vi "DCA Calibration Warning.vi"(4 "error in (no error)":errorcluster, 7 "Message (\"\")":string="The instrument does not have a normalization state consistent\nwith the measurements to be performed.  Spartan always\nrecords the instrument normalization state when test sequences\nare executed.\n\nPlease select one of the following options:\n\n    Normalize  -  run the normalization process on the instrument now\n    Ignore  -  continue without nullification\n    Abort  -  abort this test execution\n    Abort All  -  abort the entire sequence") -> (0 "error out":errorcluster, 3 "Choice":T1=enum."Ignore")   [LabVIEW 2011]
uses:
  TypeDefs/DCA Dialog Response.ctl
panel:
  in  "Abort All":bool
  in  "Abort":bool
  in  "Ignore":bool
  in  "Normalize":bool
  out "Cal Header":string="Requested Normalization State: On"
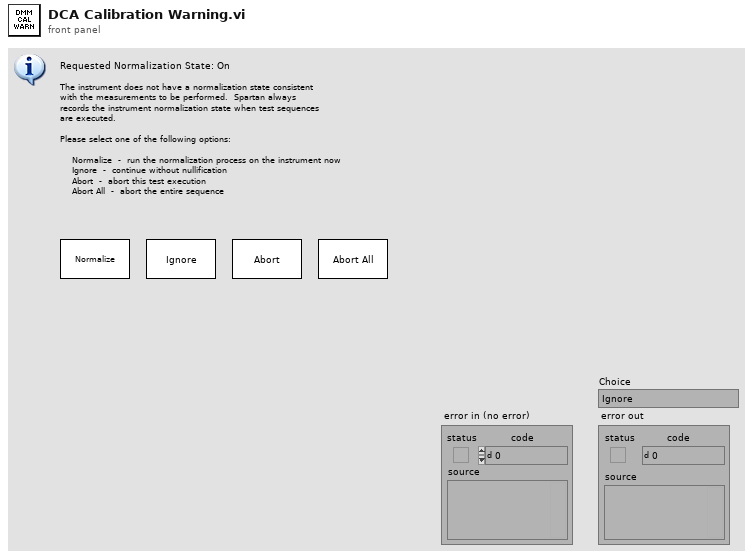
[diagram p1: front panel]
types:
  T1 = typedef "DCA Dialog Response.ctl" = enum16{"None", "Normalize", "Ignore", "Abort", "Abort All"}
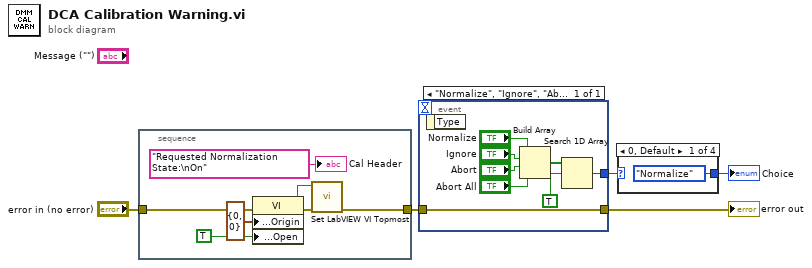
[diagram p0: block diagram]
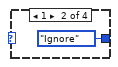
[diagram p2: hidden frame]
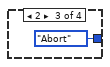
[diagram p3: hidden frame]
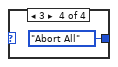
[diagram p4: hidden frame]
diagram:
  n1 = stacked-sequence {
    tunnel: "error in (no error)" -> [w12]
    tunnel: [w9] -> w3
    frame #0 {
      n2 = property on="Property Node" class="VI"(error in=w12, "Front Panel Window:Origin"=cluster{"Horizontal":i16, "Vertical":i16} {"Horizontal"=0, "Vertical"=0}, "Front Panel Window:Open"=TRUE) -> (reference out=w8:refnum<vi>, error out=w10:errorcluster)  [unwired: 1 in]
      n3 = call "Set LabVIEW VI Topmost.vi"("error in (no error)"=w10, "VI Refnum (null)"=w8) -> ("error out"=w9:errorcluster)  [unwired: 7 in, 2 out]
      "Cal Header" <- "Requested Normalization State:\nOn"
    }
  }
  n4 = event shown="[0] \"Normalize\", \"Ignore\", \"Abort\", \"Abort All\": Value Change" {
    selector: _ -> [_]
    dyn-events: _ -> [_]
    timeout: _ -> [_]
    tunnel: w3 -> [w20]
    tunnel: [w20] -> w5
    tunnel: [w14] -> w1
    event "Normalize", "Ignore", "Abort", "Abort All": Value Change {
      n5 = event-data() -> ()  [unwired: 2 out]
      n6 = Build Array("Normalize", "Ignore", "Abort", "Abort All") -> (w16:bool[])
      n7 = Search 1D Array(1D array=w16, element=TRUE) -> (index of element=w14:i32)  [unwired: 1 out]
    }
  }
  "error out" <- w5
  n8 = case shown="0, Default" w1 {
    tunnel: [DCA_Dialog_Response."Normalize" ("Action") DCA_Dialog_Response."Ignore" ("Action") DCA_Dialog_Response."Abort" ("Action") DCA_Dialog_Response."Abort All" ("Action")] -> w2
    frame 0, Default {
    }
    frame 1 {
    }
    frame 2 {
    }
    frame 3 {
    }
  }
  "Choice" <- w2
